vi "(Sub_VI)_StepSignalGen.vi"(4 "Length of Desired flow (Sec)":dbl, 6 "Sample Rate (Hz) = Bscan":dbl, 7 "Step Period(s)":dbl=20.0, 8 "#Down Steps":i32=4, 9 "#Up Steps":i32=3, 10 "Max Value":dbl=0.5, 11 "Min Value":dbl=0.1) -> (3 "Waveform Graph":dbl[](graph))   [LabVIEW 2019]
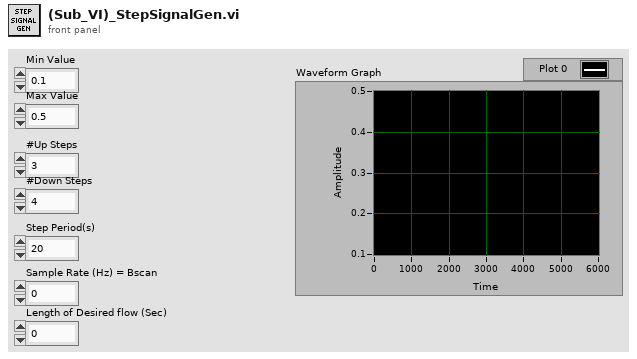
[diagram p1: front panel]
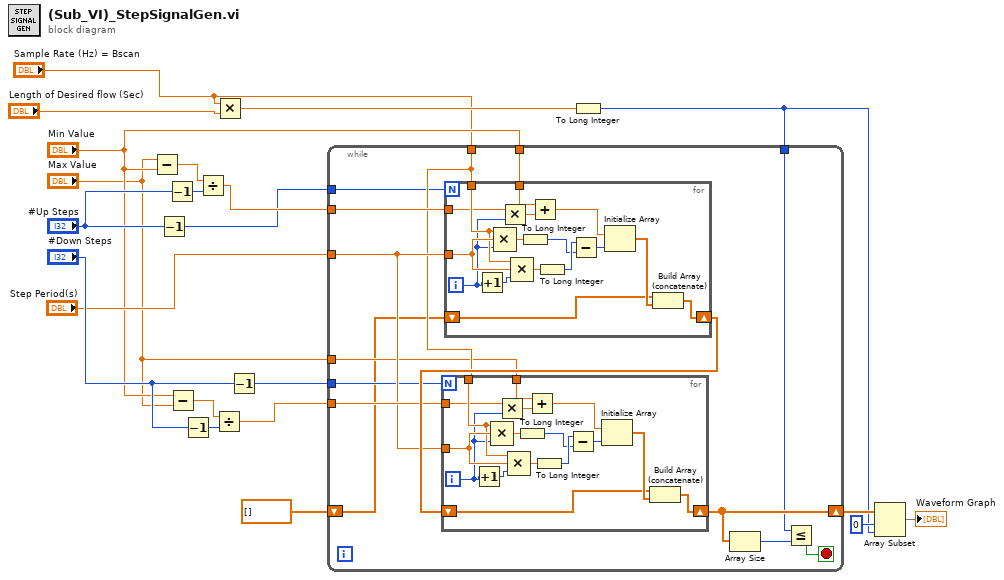
[diagram p0: block diagram]
diagram:
  n1 = Subtract(x="Max Value", y="Min Value") -> (x-y=w21:dbl)
  n2 = Decrement(x="#Up Steps") -> (x-1=w10:i32)
  n3 = Decrement(x="#Up Steps") -> (x-1=w20:i32)
  n4 = Subtract(x="Min Value", y="Max Value") -> (x-y=w16:dbl)
  n5 = Decrement(x="#Down Steps") -> (x-1=w17:i32)
  n6 = Divide(x=w21, y=w20) -> (x/y=w18:dbl)
  n7 = Divide(x=w16, y=w17) -> (x/y=w14:dbl)
  n8 = Multiply(x="Sample Rate (Hz) = Bscan", y="Length of Desired flow (Sec)") -> (x*y=w8:dbl)
  n9 = Decrement(x="#Down Steps") -> (x-1=w9:i32)
  n10 = To Long Integer(number=w8) -> (32bit integer=w4:i32)
  n11 = while {
    tunnel: w18 -> [w35]
    tunnel: w14 -> [w33]
    tunnel: "Step Period(s)" -> [w32]
    tunnel: "Sample Rate (Hz) = Bscan" -> [w31]
    tunnel: "Min Value" -> [w30]
    tunnel: "Max Value" -> [w29]
    tunnel: w10 -> [w28]
    tunnel: w9 -> [w27]
    tunnel: w4 -> [w24]
    shift-right: [w26] -> w6
    shift-left: dbl[] [] -> [w22]
    stop <- w25 stop-if-true
    n12 = for {
      N: w28 -> [_]
      tunnel: w31 -> [w63]
      tunnel: w32 -> [w64]
      tunnel: w35 -> [w59]
      tunnel: w30 -> [w56]
      shift-right: [w54] -> w34
      shift-left: w22 -> [w52]
      i -> [w58]
      n13 = Increment(x=w58) -> (x+1=w65:i32)
      n14 = Compound Arithmetic op=MULTIPLY(w63, w64, w58) -> (w66:dbl)
      n15 = Multiply(x=w59, y=w58) -> (x*y=w57:dbl)
      n16 = Compound Arithmetic op=MULTIPLY(w63, w64, w65) -> (w67:dbl)
      n17 = To Long Integer(number=w66) -> (32bit integer=w61:i32)
      n18 = Add(x=w56, y=w57) -> (x+y=w55:dbl)
      n19 = To Long Integer(number=w67) -> (32bit integer=w62:i32)
      n20 = Subtract(x=w62, y=w61) -> (x-y=w60:i32)
      n21 = Initialize Array(w55, w60) -> (w53:dbl[])
      n22 = Build Array (concatenate)(w52, w53) -> (w54:dbl[])
    }
    n23 = for {
      N: w27 -> [_]
      tunnel: w31 -> [w47]
      tunnel: w32 -> [w48]
      tunnel: w33 -> [w43]
      tunnel: w29 -> [w40]
      shift-right: [w38] -> w26
      shift-left: w34 -> [w36]
      i -> [w42]
      n24 = Increment(x=w42) -> (x+1=w49:i32)
      n25 = Compound Arithmetic op=MULTIPLY(w47, w48, w42) -> (w50:dbl)
      n26 = Multiply(x=w43, y=w42) -> (x*y=w41:dbl)
      n27 = Compound Arithmetic op=MULTIPLY(w47, w48, w49) -> (w51:dbl)
      n28 = To Long Integer(number=w50) -> (32bit integer=w45:i32)
      n29 = Add(x=w40, y=w41) -> (x+y=w39:dbl)
      n30 = To Long Integer(number=w51) -> (32bit integer=w46:i32)
      n31 = Subtract(x=w46, y=w45) -> (x-y=w44:i32)
      n32 = Initialize Array(w39, w44) -> (w37:dbl[])
      n33 = Build Array (concatenate)(w36, w37) -> (w38:dbl[])
    }
    n34 = Array Size(array=w26) -> (size(s)=w23:i32)
    n35 = Less Or Equal?(x=w24, y=w23) -> (x <= y?=w25:bool)
  }
  n36 = Array Subset(array=w6, index=0, length=w4) -> (→"Waveform Graph":dbl[])
